vi "main.vi"() -> ()   [LabVIEW 2020, in "main.lvlib"]
uses:
  main.lvlib
  <instrlib>/HH PLA Series/HH PLA Series.lvlib
panel:
  out "Waveform Chart":dbl(graph)
  out "Pmpp":dbl format="%.2f W"
  out "Impp":dbl format="%.2f A"
  out "Vmpp":dbl format="%.2f V"
  in  "Stop":bool
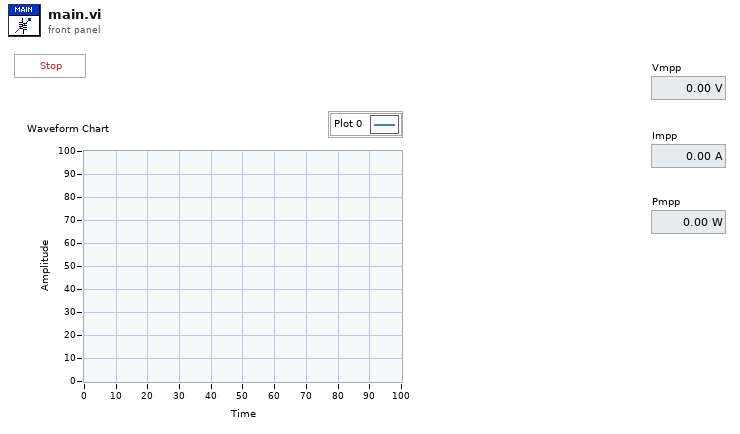
[diagram p1: front panel]
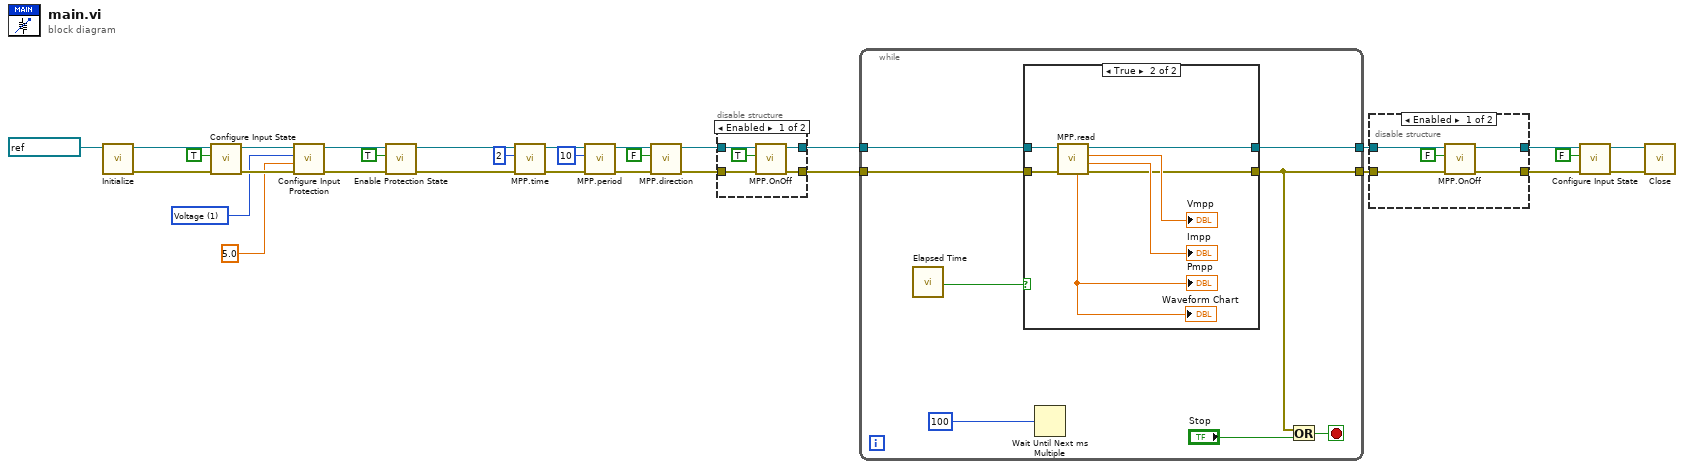
[diagram p0: block diagram]
diagram:
  w7 = u16 1 items=["Current", "Voltage"] ("Protection Mode (Current)")
  n1 = call <instrlib>:"Initialize.vi"("VISA resource name"=refnum<visa-resource-name> "PLA-HH") -> ("error out"=w16:errorcluster, "VISA resource name out"=w17:refnum<visa-resource-name>)  [unwired: 9 in]
  n2 = call <instrlib>:"Configure Input State.vi"("error in (no error)"=w16, "Input State (Off)"=TRUE, "VISA resource name"=w17) -> ("error out"=w8:errorcluster, "VISA resource name out"=w9:refnum<visa-resource-name>)  [unwired: 7 in]
  n3 = call <instrlib>:"Configure Input Protection.vi"("error in (no error)"=w8, "Protection Value (0)"=5.0, "Protection Mode (Current)"=w7, "VISA resource name"=w9) -> ("error out"=w3:errorcluster, "VISA resource name out"=w5:refnum<visa-resource-name>)  [unwired: 6 in]
  n4 = call <instrlib>:"Enable Protection State.vi"("error in (no error)"=w3, "Protection State (Off)"=TRUE, "VISA resource name"=w5) -> ("error out"=w2:errorcluster, "VISA resource name out"=w4:refnum<visa-resource-name>)  [unwired: 7 in]
  n5 = call "MPP.time.vi"("error in (no error)"=w2, "time"=u16 2, "VISA Refnum in"=w4) -> ("error out"=w26:errorcluster, "VISA Refnum out"=w27:refnum<visa-resource-name>)  [unwired: 7 in]
  n6 = call "MPP.period.vi"("error in (no error)"=w26, "time"=u16 10, "VISA Refnum in"=w27) -> ("error out"=w20:errorcluster, "VISA Refnum out"=w22:refnum<visa-resource-name>)  [unwired: 7 in]
  n7 = call "MPP.direction.vi"("error in (no error)"=w20, "UP?"=FALSE, "VISA Refnum in"=w22) -> ("error out"=w19:errorcluster, "VISA Refnum out"=w21:refnum<visa-resource-name>)  [unwired: 7 in]
  n8 = disable-structure shown="Enabled" {
    disable-tunnel: [w35 w37] -> w24
    disable-tunnel: [w34 w38] -> w23
    disable-tunnel: w21 -> [w33 w38]
    disable-tunnel: w19 -> [w32 w37]
    frame Enabled {
      n9 = call "MPP.OnOff.vi"("error in (no error)"=w32, "ON?"=TRUE, "VISA Refnum in"=w33) -> ("error out"=w35:errorcluster, "VISA Refnum out"=w34:refnum<visa-resource-name>)  [unwired: 7 in]
    }
    frame Disabled {
    }
  }
  n10 = while {
    tunnel: w23 -> [w41]
    tunnel: w24 -> [w40]
    tunnel: [w43] -> w30
    tunnel: [w42] -> w29
    stop <- w46 stop-if-true
    n11 = call "Elapsed Time"() -> ("Time has Elapsed"=w39:bool)  [unwired: 12 in, 7 out]
    n12 = case shown="True" w39 {
      tunnel: [w48 w53] -> w43
      tunnel: [w47 w52] -> w42
      tunnel: w41 -> [w48 w51]
      tunnel: w40 -> [w47 w50]
      frame False {
      }
      frame True {
        n13 = call "MPP.read.vi"("error in (no error)"=w50, "VISA Refnum in"=w51) -> ("error out"=w52:errorcluster, "Impp"=→"Impp":dbl, "Vmpp"=→"Vmpp":dbl, "VISA Refnum out"=w53:refnum<visa-resource-name>, "Pmpp"=→"Pmpp" →"Waveform Chart":dbl)  [unwired: 5 in]
      }
    }
    n14 = Wait Until Next ms Multiple(millisecond multiple=u32 100) -> ()  [unwired: 1 out]
    n15 = Or(x=w42, y="Stop") -> (x .or. y?=w46:bool)
  }
  n16 = disable-structure shown="Enabled" {
    disable-tunnel: [w59 w62] -> w13
    disable-tunnel: [w58 w61] -> w12
    disable-tunnel: w30 -> [w57 w62]
    disable-tunnel: w29 -> [w56 w61]
    frame Enabled {
      n17 = call "MPP.OnOff.vi"("error in (no error)"=w56, "ON?"=FALSE, "VISA Refnum in"=w57) -> ("error out"=w58:errorcluster, "VISA Refnum out"=w59:refnum<visa-resource-name>)  [unwired: 7 in]
    }
    frame Disabled {
    }
  }
  n18 = call <instrlib>:"Configure Input State.vi"("error in (no error)"=w12, "Input State (Off)"=FALSE, "VISA resource name"=w13) -> ("error out"=w11:errorcluster, "VISA resource name out"=w10:refnum<visa-resource-name>)  [unwired: 7 in]
  n19 = call <instrlib>:"Close.vi"("error in (no error)"=w11, "VISA resource name"=w10) -> ()  [unwired: 9 in, 1 out]
